vi "CfgGetCameraExposure.vi"(8 "error in (no error)":errorcluster, 11 "configuration file path":path) -> (0 "error out":errorcluster, 3 "cam exposure":dbl)   [LabVIEW 2019]
uses:
  <vilib>/Utility/config.llb/Read Key (Double).vi
  <vilib>/Utility/config.llb/NI_LVConfig.lvlib
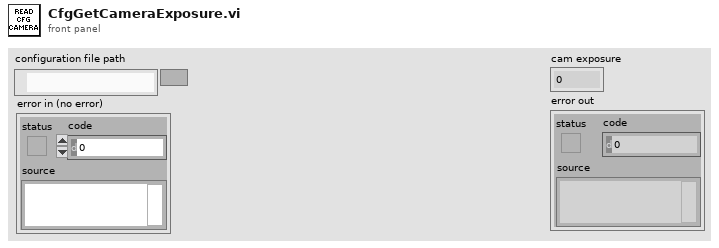
[diagram p1: front panel]
types:
  T1 = typedef "NI_LVConfig.lvlib/Config Data RefNum.ctl" = refnum<k1>
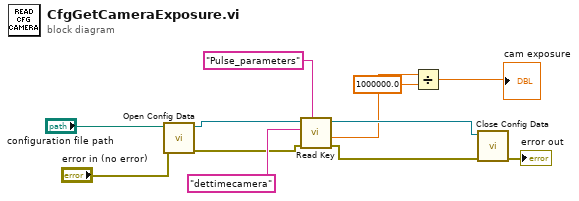
[diagram p0: block diagram]
diagram:
  n1 = call <vilib>:"Open Config Data.vi"("error in (no error)"="error in (no error)", "configuration file path"="configuration file path") -> ("error out"=w9:errorcluster, "refnum"=w11:T1)  [unwired: 7 in, 1 out]
  n2 = call-poly <vilib>:"Read Key.vi"("section"="Pulse_parameters", "error in (no error)"=w9, "key"="dettimecamera", "refnum"=w11) -> ("error out"=w8:errorcluster, "value"=w3:dbl, "refnum out"=w7:T1)  [unwired: 4 in, 1 out]
  n3 = Divide(x=w3, y=1000000.0) -> (x/y=→"cam exposure":dbl)
  n4 = call <vilib>:"Close Config Data.vi"("error in (no error)"=w8, "refnum"=w7) -> ("error out"=→"error out":errorcluster)  [unwired: 8 in, 1 out]
